vi "Obtain Message Queue.vi"(8 "error in (no error)":T1 caption="entrée d'erreur (pas d'erreur)") -> (0 "error out":T1 caption="sortie d'erreur", 3 "File d'attente de messages":refnum<queue>)   [LabVIEW 2020, in "Message Queue.lvlib"]
doc: "Créer une file d'attente avec le type de données du cluster Message."
uses:
  Message Queue.lvlib
  Message Cluster.ctl
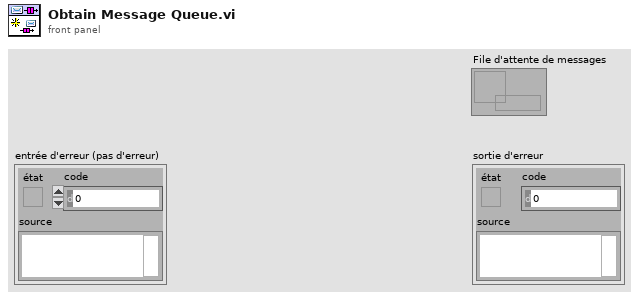
[diagram p1: front panel]
types:
  T1 = cluster{"état":bool, "code":i32, "source":string}
  T2 = typedef "Message Queue.lvlib/Message Cluster.ctl" = cluster{"Message":string, "Données de message":variant}
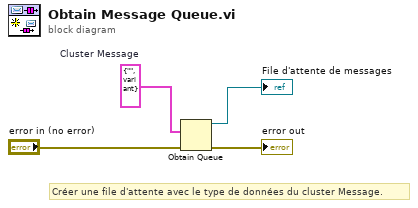
[diagram p0: block diagram]
diagram:
  w4 = T2 {"Message"="", "Données de message"=variant}  # Cluster Message
  # "Créer une file d'attente avec le type de données du cluster Message."
  n1 = Obtain Queue(element data type=w4, error in (no error)="error in (no error)") -> (queue out=→"File d'attente de messages":refnum<queue>, error out=→"error out":errorcluster)  [unwired: 3 in, 1 out]
